vi "Configure Channel.vi"(0 "device session in":refnum<class "Device Session.lvclass">, 1 "enable channel (T)":bool=TRUE, 5 "channel":u32, 7 "vertical range (Vpp)":dbl=1.0 format="%#_6p", 9 "bandwidth":T1(ring), 11 "error in":errorcluster, 12 "coupling":enum8{"Default", "DC", "AC"}(ring), 13 "impedance":enum8{"Default", "1 mega ohm", "50 ohm"}(ring)) -> (4 "device session out":refnum<class "Device Session.lvclass">, 6 "actual channel configuration":T2 {"vertical offset" format="%_3p"; "vertical range" format="%_3p"}, 15 "error out":errorcluster)   [LabVIEW 2015, in "Device Session.lvclass"]
doc: "Configures a channel with the specified parameters and uses the coerced configuration to compute the coefficients for a scaled fetch. These coefficients are stored as part of the device session.\n\n<B>Input Parameters</B>\n\n<B>enable channel (T)</B> enables or disables the channel. Setting this value to FALSE physically disconnects the channel.\n\n<B>device session in</B> is a reference to the session containing sessions to all instrument design libraries used in this sample project. This parameter is obtained from the 'Open Session' VI.\n\n<B>vertical range (Vpp)</B> specifies in volts the absolute value of the input range for the channel. The default peak-to-peak value (Vpk-pk) is 1 V.\n\n<B>channel</B> specifies the channel to be configured. The default channel is 0.\n\n<B>bandwidth</B> specifies the bandwidth configuration for the channel.\n\n'Default': The default bandwidth setting for the device.\n'Full Bandwidth': No attenuation of the signal.\n'Anti-alias Filter': Attenuates unwanted high-frequency components of an analog signal prior to its conversion into a digital value. These signals would otherwise appear as undesired, aliased frequency components.\n\n<B>coupling</B> specifies the coupling configuration for the channel.\n\n'Default': The default coupling setting of the device.\n'DC': Direct Current signal components will not be attenuated.\n'AC': Alternating Current signal components will not be attenuated.\n\n<B>impedance</B> specifies the impedance configuration for the channel.\n\n'Default': The default impedance setting for the device.\n'1 MOhm': The impedance of the channel will be configured at 1 MOhm.\n'50 Ohm': The impedance of the channel will be configured at 50 Ohms.\n\n<B>error in</B> describes error conditions that occur before this node runs. This input provides standard 'error in' functionality.\n\n<B>Output Parameters</B>\n\n<B>device session out</B> passes a reference to the session to the next VI.\n\n<B>actual channel configuration</B> returns the coerced configuration used to configure the channel.\n\n<B>actual channel configuration.channel</B> is the channel that was configured.\n\n<B>actual channel configuration.coupling</B> is the coupling configuration applied to the channel.\n\n'Default': The default coupling setting for the device.\n'DC': Direct Current coupling.\n'AC': Alternating Current coupling.\n\n<B>actual channel configuration.impedance</B> is the impedance configuration applied to the channel.\n\n'Default': The channel was configured with the default impedance setting for the device.\n'1 mega ohm': The channel was configured with 1 MOhm of impedance.\n'50 ohm': The channel was configured with 50 Ohms of impedance.\n\n<B>actual channel configuration.bandwidth</B> is the coerced bandwidth configuration applied to the channel.\n\n'Default': The default bandwidth setting for the device. The 'bandwidth' of the 'actual channel configuration' will return the actual bandwidth value.\n'Full Bandwidth': No attenuation of the signal.\n'Anti-alias Filter': Attenuates unwanted high-frequency signals of an analog signal prior to its conversion into a digital value. These signals would otherwise appear as undesired, aliased frequency components.\n\n<B>actual channel configuration.vertical range</B> is the coerced input range applied to the channel.\n\n<B>actual channel configuration.vertical offset</B> is the coerced vertical offset configuration applied to the channel.\n\n<B>error out</B> contains error information. This output provides standard 'error out' functionality."
uses:
  Device Session.lvclass
  <instrlib>/HSAI-RIO/Types/v1/Host/Typedefs/Channel Configuration.ctl
  <instrlib>/HSAI-RIO/Types/v1/Host/Typedefs/Coupling.ctl
  <instrlib>/HSAI-RIO/Types/v1/Host/Typedefs/Impedance.ctl
  <instrlib>/HSAI-RIO/Types/v1/Host/Typedefs/Bandwidth.ctl
  Device Session.lvclass/Device Session.ctl
  <instrlib>/HSAI-RIO/Types/v1/Host/Typedefs/Additional Channel Configuration.ctl
  <instrlib>/HSAI-RIO/Config/Interface/v1/Host/niHSAI Config v1 Host.lvclass
  <instrlib>/HSAI-RIO/Types/v1/Host/niHSAI Types v1 Host.lvlib
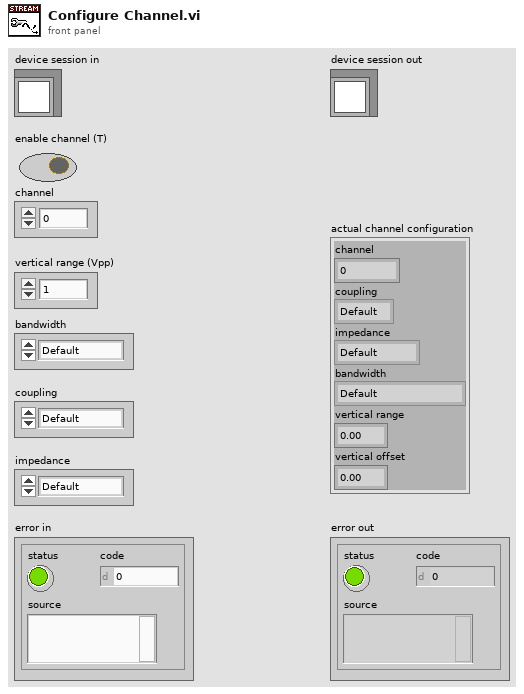
[diagram p1: front panel]
types:
  T1 = enum8{"Default", "Full Bandwidth", "Anti-alias Filter"}
  T2 = typedef "niHSAI Types v1 Host.lvlib/Channel Configuration.ctl" = cluster{"channel":u32, "coupling":T3, "impedance":T4, "bandwidth":T5, "vertical range":dbl, "vertical offset":dbl}
  T3 = typedef "niHSAI Types v1 Host.lvlib/Coupling.ctl" = enum8{"Default", "DC", "AC"}
  T4 = typedef "niHSAI Types v1 Host.lvlib/Impedance.ctl" = enum8{"Default", "1 mega ohm", "50 ohm"}
  T5 = typedef "niHSAI Types v1 Host.lvlib/Bandwidth.ctl" = enum8{"Default", "Full Bandwidth", "Anti-alias Filter"}
  T6 = typedef "niHSAI Types v1 Host.lvlib/Additional Channel Configuration.ctl" = cluster{"Bandwidth":T5, "Coupling":T3, "Impedance":T4}
  T7 = typedef "Device Session.lvclass/Device Session Object.ctl" = cluster{"ni5171R FPGA Reference":T8, "niHSAI config":refnum<class "niHSAI Config v1 Host.lvclass">, "configured scaling coefficients":cluster{"gain":dbl, "offset":dbl}[], "number of channels to stream":u8, "selected acq channels":bool[], "number of channels":u32, "actual channel configuration":T2[], "configured channels":bool[], "sample clock rate (Hz)":dbl}
  T8 = typedef "Device Session.lvclass/FPGA Refnum.ctl" = refnum<k20>
  T9 = typedef "niHSAI Types v1 Host.lvlib/Scaling Coefficients.ctl" = cluster{"gain":dbl, "offset":dbl}
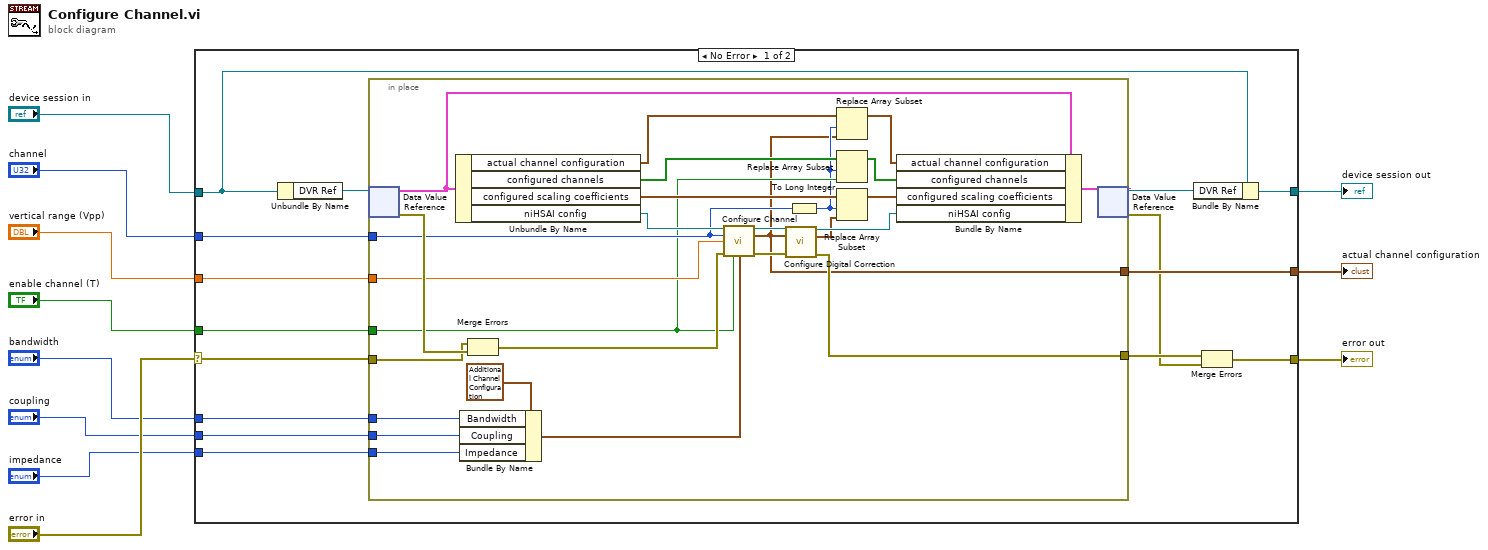
[diagram p0: block diagram]
diagram:
  n1 = case shown="No Error" "error in" {
    selector: "error in" -> [w24 w55]
    tunnel: "device session in" -> [w20 w54]
    tunnel: [w19 w54] -> w9
    tunnel: "enable channel (T)" -> [w26 _]
    tunnel: "vertical range (Vpp)" -> [w25 _]
    tunnel: [w23 _] -> w4
    tunnel: [w18 w55] -> w6
    tunnel: "channel" -> [w17 _]
    tunnel: "bandwidth" -> [w14 _]
    tunnel: "coupling" -> [w13 _]
    tunnel: "impedance" -> [w12 _]
    frame No Error {
      n2 = Unbundle By Name(w20) -> ("DVR Ref"=w22:refnum<data-value>)
      n3 = in-place {
        in-place-border: w26 -> [w32]
        in-place-border: w25 -> [w48]
        in-place-border: w24 -> [w49]
        in-place-border: [w27] -> w23
        in-place-border: [w40] -> w16
        in-place-border: w17 -> [w34]
        in-place-border: w14 -> [w45]
        in-place-border: w13 -> [w44]
        in-place-border: w12 -> [w43]
        n4 = in-place-dvr #1(w22) -> (w53:T7, w51:errorcluster)
        n5 = Unbundle By Name(w53) -> ("actual channel configuration"=w29:T2[], "configured channels"=w33:bool[], "configured scaling coefficients"=w37:cluster{"gain":dbl, "offset":dbl}[], "niHSAI config"=w38:refnum<class "niHSAI Config v1 Host.lvclass">)
        n6 = Bundle By Name(cluster=T6 {"Bandwidth"=enum."Default", "Coupling"=enum."Default", "Impedance"=enum."Default"} ("additional channel configuration"), "Bandwidth"=w45, "Coupling"=w44, "Impedance"=w43) -> (w46:T6)
        n7 = Merge Errors(w49, w51) -> (w50:errorcluster)
        n8 = call-dynamic "Configure Channel.vi"("session in"=w38, "channel"=w34, "vertical range (V)"=w48, "error in"=w50, "enable channel (T)"=w32, "additional channel configuration"=w46) -> ("session out"=w42:refnum<class "niHSAI Config v1 Host.lvclass">, "actual channel configuration"=w27:T2, "error out"=w39:errorcluster)  [unwired: 6 in, 1 out]
        n9 = call-dynamic "Configure Digital Correction.vi"("session in"=w42, "actual channel configuration"=w27, "error in"=w39) -> ("session out"=w41:refnum<class "niHSAI Config v1 Host.lvclass">, "scaling coefficients"=w35:T9, "error out"=w40:errorcluster)  [unwired: 10 in]
        n10 = To Long Integer(number=w34) -> (32bit integer=w30:i32)
        n11 = Replace Array Subset(array=w29, new element=w27, index=w30) -> (w28:T2[])
        n12 = Replace Array Subset(array=w33, new element=w32, index=w30) -> (w31:bool[])
        n13 = Replace Array Subset(array=w37, new element=w35, index=w30) -> (w36:cluster{"gain":dbl, "offset":dbl}[])
        n14 = Bundle By Name(cluster=w53, "actual channel configuration"=w28, "configured channels"=w31, "configured scaling coefficients"=w36, "niHSAI config"=w41) -> (w52:T7)
        n15 = in-place-dvr #1(w52) -> (w21:refnum<data-value>, w15:errorcluster)
      }
      n16 = Bundle By Name(cluster=w20, "DVR Ref"=w21) -> (w19:refnum<class "Device Session.lvclass">)
      n17 = Merge Errors(w16, w15) -> (w18:errorcluster)
    }
    frame Error {
    }
  }
  "error out" <- w6
  "device session out" <- w9
  "actual channel configuration" <- w4
